vi "Get All Menu Items.vi"(8 "error in (no error)":errorcluster, 10 "Item Tags (Default: All)":string[](array[string])=[""], 11 "Menu in":refnum<k9>) -> (0 "error out":errorcluster, 2 "All Menu Tags":string[](array[string]), 3 "Menu out":refnum<k9>)   [LabVIEW 2021, in "Menu.lvlib"]
doc: "This VI returns all menu tags below the provided top menu items (recursively).\n\nThe 'APP_SEPARATOR' tags are removed, as well as the top menu tag (an empty string).\n\nTo obtain all tabs in a menu, do not wire the <B>Item Tags</B> input."
uses:
  Menu.lvlib
  9b585f0a-4a06-4b47-8853-1520955bd0fa.vi
  <userlib>/_OpenG.lib/array/array.llb/Filter 1D Array (String)__ogtk.vi
  <userlib>/_OpenG.lib/array/array.llb/openg_array.lvlib
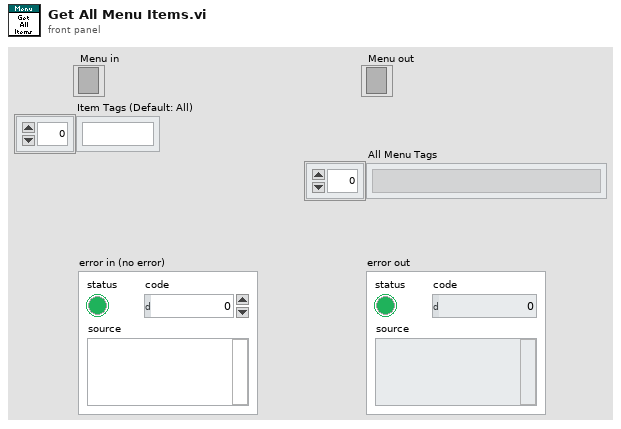
[diagram p1: front panel]
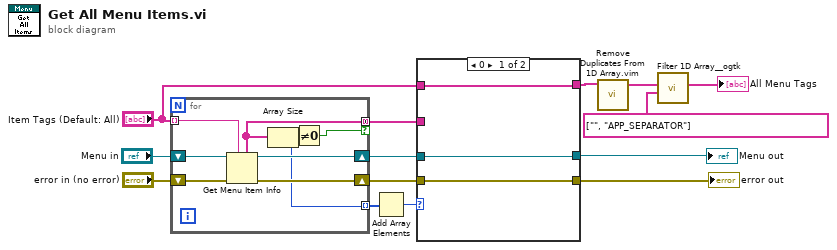
[diagram p0: block diagram]
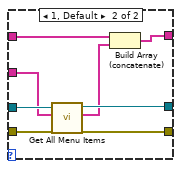
[diagram p2: hidden frame]
diagram:
  n1 = for {
    tunnel: [w17] -> w8 mode=concatenating if=w16
    tunnel: "Item Tags (Default: All)" -> [w18] mode=indexing
    shift-right: [w22] -> w11
    shift-left: "error in (no error)" -> [w21]
    shift-right: [w20] -> w12
    shift-left: "Menu in" -> [w19]
    tunnel: [w15] -> w5 mode=indexing
    n2 = Get Menu Item Info(7:w18, 8:w21, 11:w19) -> (0:w22:errorcluster, 3:w20:refnum<k9>, 5:w17:string[])  [unwired: 4 out]
    n3 = Array Size(array=w17) -> (size(s)=w15:i32)
    n4 = Not Equal To 0?(x=w15) -> (x != 0?=w16:bool)
  }
  n5 = Add Array Elements(numeric array=w5) -> (sum=w4:i32)
  n6 = case shown="0" w4 {
    tunnel: w12 -> [w24 w33]
    tunnel: w11 -> [w23 w32]
    tunnel: [w24 w31] -> w10
    tunnel: [w23 w30] -> w9
    tunnel: w8 -> [_ w29]
    tunnel: "Item Tags (Default: All)" -> [w25 w27]
    tunnel: [w25 w26] -> w6
    frame 0 {
    }
    frame 1, Default {
      n7 = call "Get All Menu Items.vi"("error in (no error)"=w32, "Item Tags (Default: All)"=w29, "Menu in"=w33) -> ("error out"=w30:errorcluster, "All Menu Tags"=w28:string[], "Menu out"=w31:refnum<k9>)  [unwired: 6 in]
      n8 = Build Array (concatenate)(w27, w28) -> (w26:string[])
    }
  }
  "error out" <- w9
  "Menu out" <- w10
  n9 = call "Remove Duplicates From 1D Array.vim"("array"=w6) -> ("array with duplicates removed"=w3:string[])  [unwired: 10 in]
  n10 = call-poly <userlib>:"Filter 1D Array__ogtk.vi"("items to filter"=string[] ["", "APP_SEPARATOR"] ("Item Tags"), "array"=w3) -> ("filtered array"=→"All Menu Tags":string[])  [unwired: 4 in, 1 out]
